vi "Lookup Cookie Value.vi"(8 "error in (no error)":errorcluster, 10 "Name":string, 11 "Request in":refnum<class "Request.lvclass">) -> (0 "error out":errorcluster, 1 "Not Found?":bool, 2 "Value":string, 3 "Request out":refnum<class "Request.lvclass">)   [LabVIEW 2020, in "HTTP Utils.lvlib" / "Request.lvclass"]
uses:
  Request.lvclass
  Cookie/Cookie.lvclass
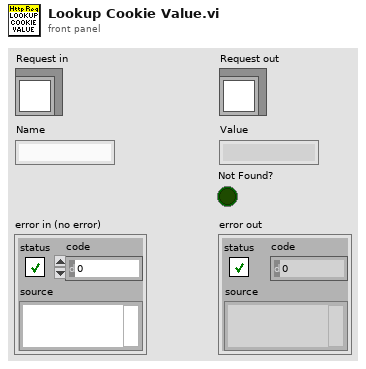
[diagram p1: front panel]
types:
  T1 = typedef "HTTP Utils.lvlib/Cookie Map.ctl" = map{string, refnum<class "Cookie.lvclass">}
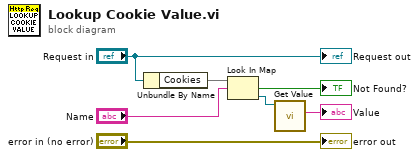
[diagram p0: block diagram]
diagram:
  n1 = Unbundle By Name("Request in") -> ("Cookies"=w5:T1)
  n2 = Look In Map(map=w5, key="Name") -> (key not found?=→"Not Found?":bool, value=w2:refnum<class "Cookie.lvclass">)  [unwired: 1 in]
  n3 = call "Get Value.vi"("Cookie in"=w2) -> ("Value"=→"Value":string)  [unwired: 8 in, 2 out]
  "error out" <- "error in (no error)"
  "Request out" <- "Request in"
